vi "Test 5 Example Data 1.vi"(8 "error in (no error)":errorcluster, 11 "Test Case In":refnum<class "Tests Rev2.lvclass">) -> (0 "error out":errorcluster, 3 "Test Case Out":refnum<class "Tests Rev2.lvclass">)   [LabVIEW 2021, in "Tests Rev2.lvclass"]
uses:
  Tests Rev2.lvclass
  C:/Program Files (x86)/National Instruments/LabVIEW 2021/vi.lib/Astemes/LUnit/Test Case.lvclass
  <vilib>/Astemes/LUnit/Test Case.lvclass/Test Case.ctl
  4993e8ee-a06a-463a-9684-69129f64d5ce.vi
  <vilib>/Astemes/LUnit/Append Pass Result.vi
  <vilib>/Astemes/LUnit/Append Fail Result.vi
  <vilib>/Astemes/LUnit/Describe Comparison.vi
  <vilib>/Astemes/LUnit/Compare Variants.vi
  <vilib>/Astemes/LUnit/Variant to string.vi
  <vilib>/Utility/Data Type/Get Type Information.vi
  <vilib>/Utility/LVClass/Get LV Class Name.vi
  Proto/Group.lvclass
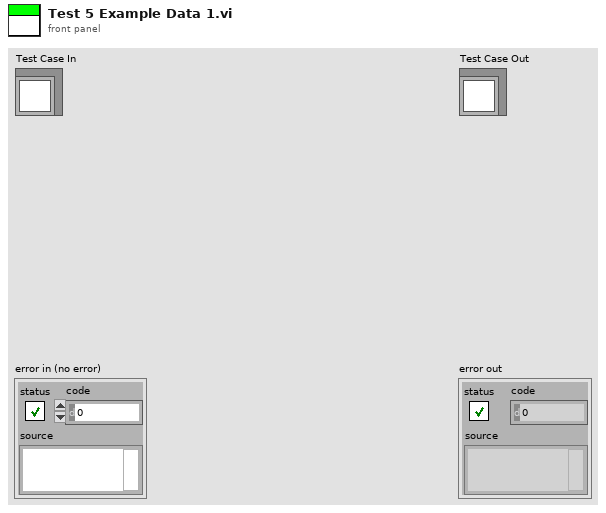
[diagram p1: front panel]
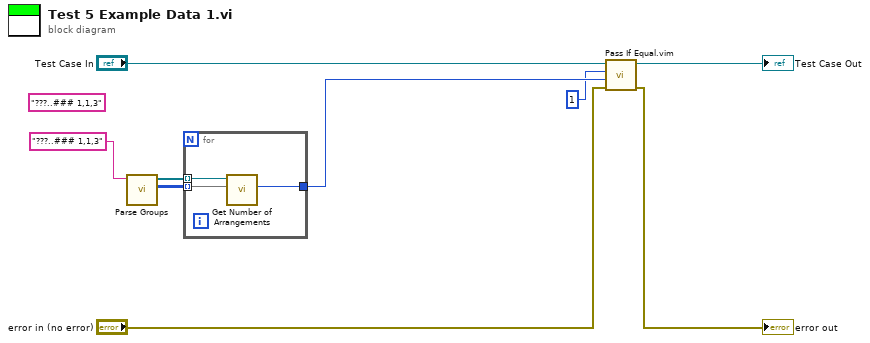
[diagram p0: block diagram]
diagram:
  (unwired) "???..### 1,1,3" ("Input")
  n1 = call "Parse Groups.vi"("Input"="???..### 1,1,3") -> ("Counts"=w2:i64[][], "Groups"=w3:refnum<class "Group.lvclass">[])  [unwired: 9 in]
  n2 = for {
    tunnel: [w12] -> w5
    tunnel: w3 -> [w11] mode=indexing
    tunnel: w2 -> [w10] mode=indexing
    n3 = call "Get Number of Arrangements.vi"("Group Sizes"=w10, "Proto in"=w11) -> ("Arrangements"=w12:u64)  [unwired: 7 in, 2 out]
  }
  n4 = call "Pass If Equal.vim"("error in (no error)"="error in (no error)", "Actual"=w5, "Expected"=u64 1 ("Arrangements"), "LUnit Test Case In"="Test Case In") -> ("error out"=→"error out":errorcluster, "LUnit Test Case Out"=→"Test Case Out":refnum<class "Tests Rev2.lvclass">)  [unwired: 6 in]
